vi "Get SubPanel.vi"(8 "error in (no error)":errorcluster, 11 "Panel in":refnum<class "Panel.lvclass">) -> (0 "error out":errorcluster, 2 "SubPanel":refnum<vi>, 3 "Panel out":refnum<class "Panel.lvclass">)   [LabVIEW 2020, in "OOPanel.lvlib" / "Panel.lvclass"]
uses:
  Panel.lvclass
  Panel.lvclass/Panel.ctl
  <vilib>/ErrorRing/Error Ring.xnode
  <vilib>/Utility/error.llb/Error Cluster From Error Code.vi
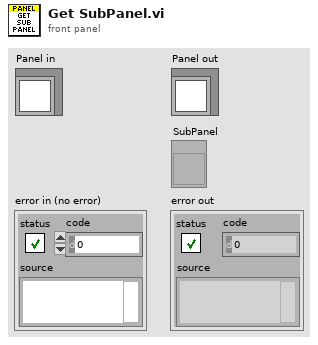
[diagram p1: front panel]
types:
  T1 = typedef "OOPanel.lvlib/Panel.lvclass/Ref Data.ctl" = cluster{"Panel Ref":refnum<vi>, "SubPanel":refnum<vi>, "Close":bool, "Running":bool, "State":T2}
  T2 = typedef "OOPanel.lvlib/Visibility State.ctl" = enum16{"Idle", "Closed", "Hidden", "Visible", "Subpanel", "Hidden Subpanel"}
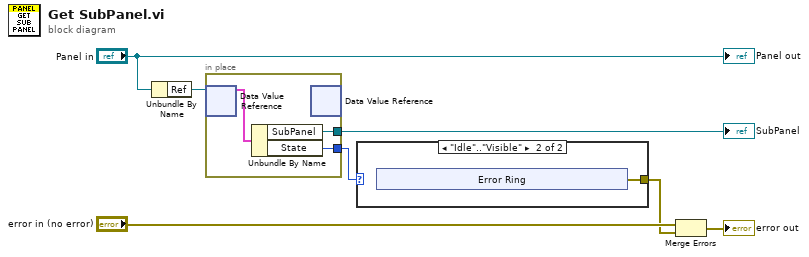
[diagram p0: block diagram]
diagram:
  n1 = Unbundle By Name("Panel in") -> ("Ref"=w6:refnum<data-value>)
  n2 = in-place {
    in-place-border: [w9] -> w4
    in-place-border: [w8] -> w2
    n3 = in-place-dvr #1(w6) -> (w10:T1)  [unwired: 1 out]
    n4 = Unbundle By Name(w10) -> ("SubPanel"=w9:refnum<vi>, "State"=w8:T2)
    n5 = in-place-dvr #1() -> ()  [unwired: 1 in, 2 out]
  }
  "SubPanel" <- w4
  n6 = case shown="\"Idle\"..\"Visible\"" w2 {
    tunnel: [_ w11] -> w1
    frame "Subpanel", "Hidden Subpanel" {
    }
    frame "Idle".."Visible" {
      n7 = xnode "Error Ring"() -> ("error out"=w11:errorcluster)
    }
  }
  n8 = Merge Errors("error in (no error)", w1) -> (→"error out":errorcluster)
  "Panel out" <- "Panel in"
